vi "dropdown2.vi"(0 "side":enum16{"l", "r"}(ring), 1 "Boolean":bool) -> ()   [LabVIEW 2017]
uses:
  <vilib>/myRIO/Instrument Drivers/Onboard IO/DIO/typedefs/DIO Reference.ctl
  <vilib>/myRIO/Common/Instrument Driver Framework/Utilities/typedefs/myRIO Generic Hardware Reference.ctl
  <vilib>/myRIO/Common/Instrument Driver Framework/Utilities/typedefs/Hardware Version Enum.ctl
  <vilib>/myRIO/Common/Instrument Driver Framework/Utilities/typedefs/myRIO v1.0 Reference.ctl
  <vilib>/myRIO/Common/Instrument Driver Framework/Utilities/typedefs/Generic FPGA Reference.ctl
  <vilib>/myRIO/Common/Instrument Driver Framework/myRIO v1.0/DIO/typedefs/DIO Channels List.ctl
  <vilib>/myRIO/Common/Instrument Driver Framework/myRIO v1.0/DIO/typedefs/DIO Channels Enum.ctl
  <vilib>/userdefined/High Color/nirio_resource_hc.ctl
  <vilib>/myRIO/Common/Instrument Driver Framework/Utilities/vis/Is FPGA Ref Available.vi
  <vilib>/myRIO/Common/Instrument Driver Framework/myRIO v1.0/DIO/vis/myRIO v1.1 Open DIO.vi
  <vilib>/myRIO/Instrument Drivers/Onboard IO/DIO/vis/Read.vi
  <vilib>/myRIO/Common/Instrument Driver Framework/Utilities/vis/Validate Channels.vi
  <vilib>/myRIO/Common/Instrument Driver Framework/myRIO v1.0/DIO/vis/myRIO v1.0 Reserve DIO.vi
  <vilib>/myRIO/Common/Instrument Driver Framework/myRIO v1.0/Resource Manager/vis/myRIO v1.0 Reserve Channel List.vi
  <vilib>/myRIO/Common/Instrument Driver Framework/myRIO v1.0/DIO/vis/myRIO v1.0 Build MUX Configuration DIO.vi
  <vilib>/myRIO/Common/Instrument Driver Framework/myRIO v1.0/Resource Manager/vis/myRIO v1.0 Reserve Channel.vi
  <vilib>/myRIO/Common/Instrument Driver Framework/myRIO v1.0/Resource Manager/vis/myRIO v1.0 Unreserve Channel.vi
  <vilib>/myRIO/Common/Instrument Driver Framework/myRIO v1.0/Resource Manager/vis/myRIO v1.0 Create Configuration List.vi
  <vilib>/myRIO/Common/Instrument Driver Framework/myRIO v1.0/Resource Manager/vis/myRIO v1.0 Build Mutex Name.vi
  <vilib>/Utility/VariantDataType/GetNumericInfo.vi
  <vilib>/Utility/error.llb/Error Cluster From Error Code.vi
  <vilib>/myRIO/Common/Instrument Driver Framework/myRIO v1.0/myRIO v1.1 Open.vi
  <vilib>/myRIO/Common/Instrument Driver Framework/Utilities/vis/IO Manager.vi
  <vilib>/myRIO/Common/Instrument Driver Framework/Utilities/vis/Configuration Manager.vi
  <vilib>/myRIO/Common/Instrument Driver Framework/myRIO v1.0/Resource Manager/vis/myRIO v1.0 Configure IO.vi
  <vilib>/myRIO/Common/Instrument Driver Framework/myRIO v1.0/myRIO v1.0 Close.vi
  <vilib>/myRIO/Common/Instrument Driver Framework/myRIO v1.0/DIO/vis/myRIO v1.0 Read DIO.vi
  <vilib>/myRIO/Express VI/Onboard IO/DI/DI Express VI.xnode
  <vilib>/myRIO/Instrument Drivers/Onboard IO/DIO/vis/myRIO DIO Open.xnode
  <vilib>/myRIO/Instrument Drivers/Onboard IO/DIO/DIO.lvlib
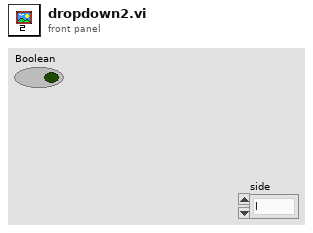
[diagram p1: front panel]
types:
  T1 = enum16{"hold", "f", "fl", "fr", "l", "r", "b", "bl", "br"}
  T2 = typedef "DIO.lvlib/DIO Reference.ctl" = cluster{"myRIO Reference":T3, "DIO Channels List":T7}
  T3 = typedef "myRIO Generic Hardware Reference.ctl" = cluster{"myRIO Model":T4, "myRIO Hardware Reference":T5}
  T4 = typedef "Hardware Version Enum.ctl" = enum16{"Unknown", "myRIO-1900", "myRIO-1950", "roboRIO", "NI ELVIS RIO CM"}
  T5 = typedef "myRIO v1.0 Reference.ctl" = cluster{"Generic FPGA Reference":T6, "Allow multiple opens":bool}
  T6 = typedef "Generic FPGA Reference.ctl" = refnum<k20>
  T7 = typedef "DIO Channels List.ctl" = T8[]
  T8 = typedef "DIO Channels Enum.ctl" = enum16{"Not Connected", "C/DIO0", "C/DIO1", "C/DIO2", "C/DIO3", "C/DIO4", "C/DIO5", "C/DIO6", "C/DIO7", "A/DIO0", "A/DIO1", "A/DIO2", "A/DIO3", "A/DIO4", "A/DIO5", "A/DIO6", "A/DIO7", "A/DIO8", "A/DIO9", "A/DIO10", "A/DIO11", "A/DIO12", "A/DIO13", "A/DIO14", "A/DIO15", "B/DIO0", "B/DIO1", "B/DIO2", "B/DIO3", "B/DIO4", "B/DIO5", "B/DIO6", "B/DIO7", "B/DIO8", "B/DIO9", "B/DIO10", "B/DIO11", "B/DIO12", "B/DIO13", "B/DIO14", "B/DIO15", "LED0", "LED1", "LED2", "LED3", "Button0", "DIO/DIO0", "DIO/DIO1", "DIO/DIO2", "DIO/DIO3", "DIO/DIO4", "DIO/DIO5", "DIO/DIO6", "DIO/DIO7", "DIO/DIO8", "DIO/DIO9", "SPI/CS0", "SPI/CS1", "SPI/CS2", "SPI/CS3", "LED RADIO (Green)", "LED RADIO (Red)", "LED COMM (Green)", "LED COMM (Red)", "LED MODE (Green)", "LED MODE (Red)"}
  T9 = typedef "nirio_resource_hc.ctl" = tag
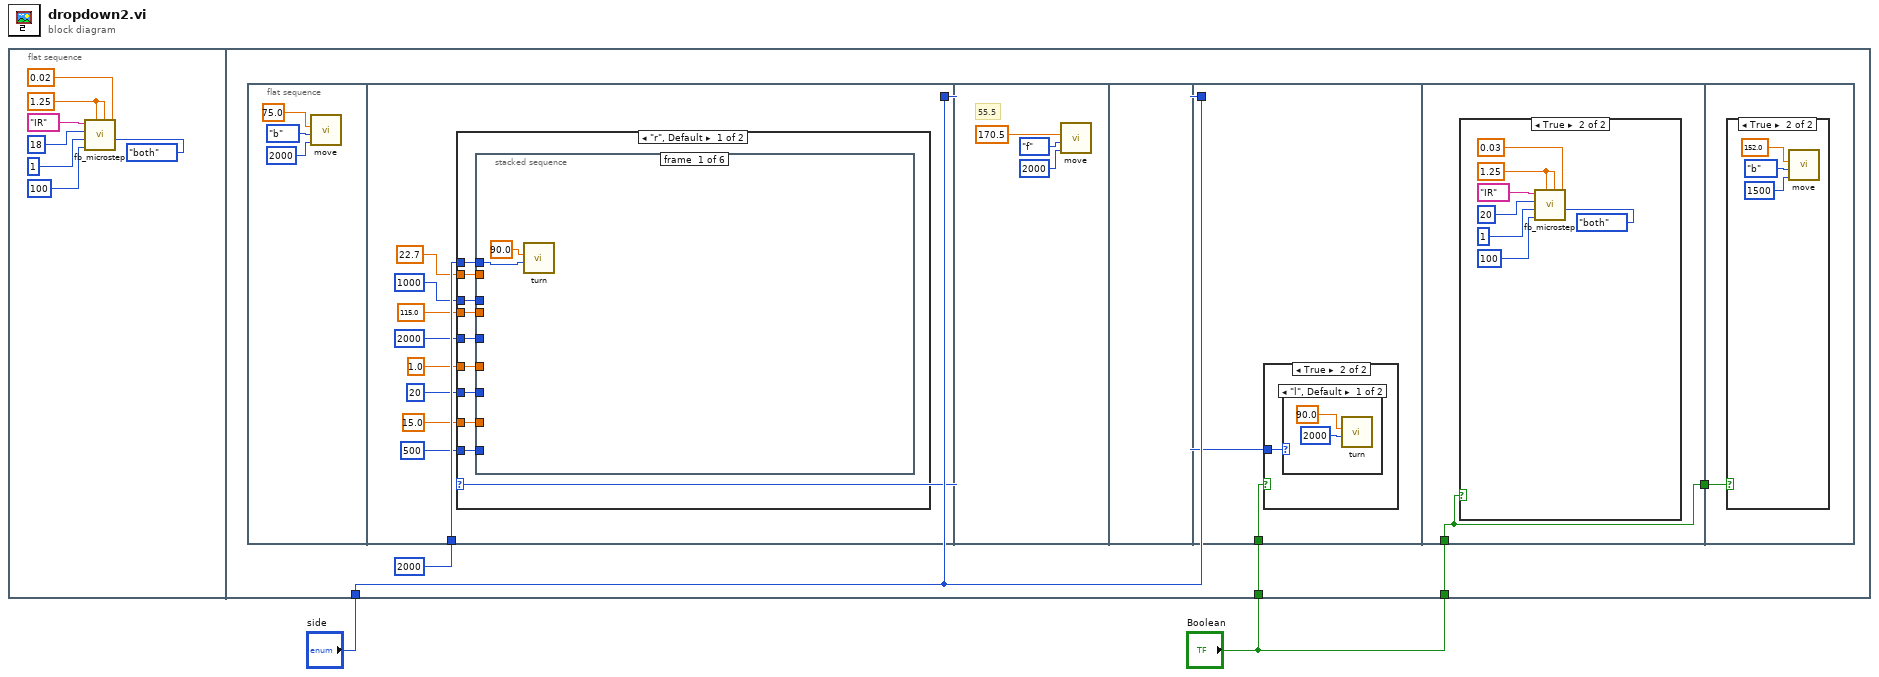
[diagram p0: block diagram]
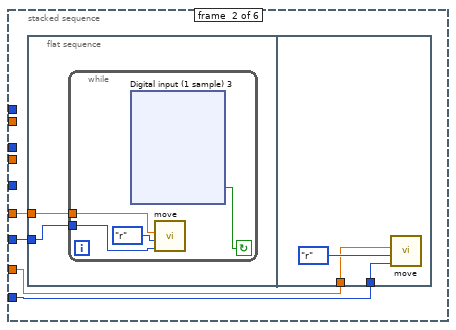
[diagram p2: hidden frame]
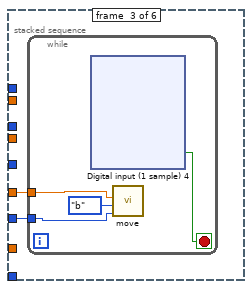
[diagram p3: hidden frame]
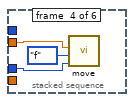
[diagram p4: hidden frame]
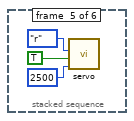
[diagram p5: hidden frame]
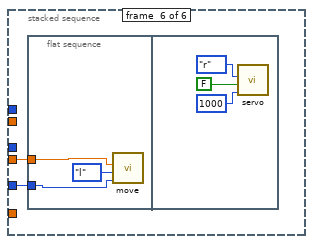
[diagram p6: hidden frame]
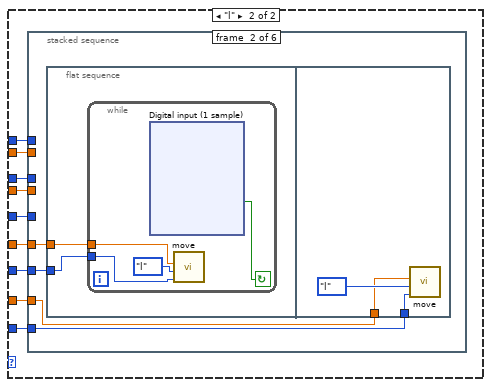
[diagram p7: hidden frame]
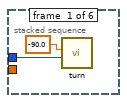
[diagram p8: hidden frame]
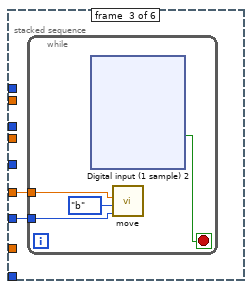
[diagram p9: hidden frame]
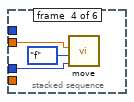
[diagram p10: hidden frame]
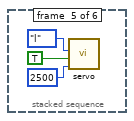
[diagram p11: hidden frame]
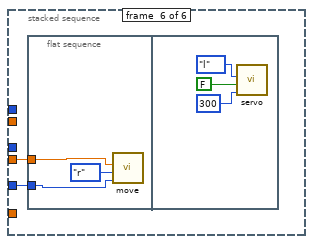
[diagram p12: hidden frame]
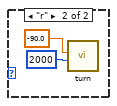
[diagram p14: hidden frame]
diagram:
  n1 = flat-sequence {
    tunnel: "side" -> [w13]
    tunnel: "Boolean" -> [w11]
    tunnel: "Boolean" -> [w10]
    frame #0 {
      w3 = 1.25 ("taget_IR_R")
      n2 = call "fb_microstep.vi"("Sensor"=enum16{"l", "r", "both"}."both", "precision"=0.02, "taget_IR_L"=w3, "taget_IR_R"=w3, "SamplingNUM"=100, "Step"=1, "Delay"=18, "Stop Mode"="IR") -> ()  [unwired: 3 in, 1 out]
    }
    frame #1 {
      n3 = flat-sequence {
        tunnel: w13 -> [w27]
        tunnel: u32 2000 ("delay") -> [w26]
        tunnel: w13 -> [w264]
        tunnel: w10 -> [w263]
        tunnel: [w270] -> w12
        tunnel: w11 -> [w270]
        tunnel: w12 -> [w278]
        frame #0 {
          n4 = call "move.vi"("delay"=u32 2000, "Enum"=T1."b", "D"=75.0) -> ()  [unwired: 9 in]
        }
        frame #1 {
          n5 = case shown="\"r\", Default" w27 {
            tunnel: w26 -> [w36 w152]
            tunnel: u32 20 ("delay") -> [w34 w151]
            tunnel: 1.0 ("D") -> [w35 w150]
            tunnel: 15.0 ("D") -> [w32 w149]
            tunnel: u32 500 ("delay") -> [w33 w148]
            tunnel: 22.7 ("D") -> [w31 w147]
            tunnel: u32 1000 ("delay") -> [w30 w146]
            tunnel: 115.0 ("D") -> [w29 w145]
            tunnel: u32 2000 ("delay") -> [w28 w144]
            frame "r", Default {
              n6 = stacked-sequence {
                tunnel: w36 -> [w37 _ _ _ _ _]
                tunnel: w35 -> [_ w42 w89 _ _ _]
                tunnel: w34 -> [_ w41 w88 _ _ _]
                tunnel: w33 -> [_ w40 _ _ _ _]
                tunnel: w32 -> [_ w39 _ _ _ _]
                tunnel: w31 -> [_ _ _ w131 _ _]
                tunnel: w30 -> [_ _ _ w130 _ _]
                tunnel: w29 -> [_ _ _ _ _ w137]
                tunnel: w28 -> [_ _ _ _ _ w136]
                frame #0 {
                  n7 = call "turn.vi"("delay"=w37, "Carzeta"=90.0) -> ()  [unwired: 10 in]
                }
                frame #1 {
                  n8 = flat-sequence {
                    tunnel: w42 -> [w44]
                    tunnel: w41 -> [w43]
                    tunnel: w40 -> [w86]
                    tunnel: w39 -> [w85]
                    frame #0 {
                      n9 = while {
                        tunnel: w44 -> [w47]
                        tunnel: w43 -> [w46]
                        stop <- w45 continue-if-true
                        n10 = xnode "Digital input (1 sample) 3"() -> ("R (A/DIO1 (Pin 13))"=w45:bool)  [unwired: 1 in, 2 out]
                        n11 = call "move.vi"("delay"=w46, "Enum"=T1."r", "D"=w47) -> ()  [unwired: 9 in]
                      }
                    }
                    frame #1 {
                      n12 = call "move.vi"("delay"=w86, "Enum"=T1."r", "D"=w85) -> ()  [unwired: 9 in]
                    }
                  }
                }
                frame #2 {
                  n13 = while {
                    tunnel: w89 -> [w92]
                    tunnel: w88 -> [w91]
                    stop <- w90 stop-if-true
                    n14 = xnode "Digital input (1 sample) 4"() -> ("R (A/DIO1 (Pin 13))"=w90:bool)  [unwired: 1 in, 2 out]
                    n15 = call "move.vi"("delay"=w91, "Enum"=T1."b", "D"=w92) -> ()  [unwired: 9 in]
                  }
                }
                frame #3 {
                  n16 = call "move.vi"("delay"=w130, "Enum"=T1."f", "D"=w131) -> ()  [unwired: 9 in]
                }
                frame #4 {
                  n17 = call "servo.vi"("delay"=u32 2500, "in=true\nout = false"=TRUE ("in=true\nout = false"), "left-right"=enum16{"r", "l"}."r") -> ()  [unwired: 9 in]
                }
                frame #5 {
                  n18 = flat-sequence {
                    tunnel: w137 -> [w139]
                    tunnel: w136 -> [w138]
                    frame #0 {
                      n19 = call "move.vi"("delay"=w138, "Enum"=T1."l", "D"=w139) -> ()  [unwired: 9 in]
                    }
                    frame #1 {
                      n20 = call "servo.vi"("delay"=u32 1000, "in=true\nout = false"=FALSE ("in=true\nout = false"), "left-right"=enum16{"r", "l"}."r") -> ()  [unwired: 9 in]
                    }
                  }
                }
              }
            }
            frame "l" {
              n21 = stacked-sequence {
                tunnel: w152 -> [w153 _ _ _ _ _]
                tunnel: w151 -> [_ w158 w205 _ _ _]
                tunnel: w150 -> [_ w157 w204 _ _ _]
                tunnel: w149 -> [_ w156 _ _ _ _]
                tunnel: w148 -> [_ w155 _ _ _ _]
                tunnel: w147 -> [_ _ _ w247 _ _]
                tunnel: w146 -> [_ _ _ w246 _ _]
                tunnel: w145 -> [_ _ _ _ _ w253]
                tunnel: w144 -> [_ _ _ _ _ w252]
                frame #0 {
                  n22 = call "turn.vi"("delay"=w153, "Carzeta"=-90.0) -> ()  [unwired: 10 in]
                }
                frame #1 {
                  n23 = flat-sequence {
                    tunnel: w158 -> [w160]
                    tunnel: w157 -> [w159]
                    tunnel: w156 -> [w202]
                    tunnel: w155 -> [w201]
                    frame #0 {
                      n24 = while {
                        tunnel: w160 -> [w162]
                        tunnel: w159 -> [w161]
                        stop <- w163 continue-if-true
                        n25 = xnode "Digital input (1 sample)"() -> ("L (A/DIO0 (Pin 11))"=w163:bool)  [unwired: 1 in, 2 out]
                        n26 = call "move.vi"("delay"=w162, "Enum"=T1."l", "D"=w161) -> ()  [unwired: 9 in]
                      }
                    }
                    frame #1 {
                      n27 = call "move.vi"("delay"=w201, "Enum"=T1."l", "D"=w202) -> ()  [unwired: 9 in]
                    }
                  }
                }
                frame #2 {
                  n28 = while {
                    tunnel: w205 -> [w207]
                    tunnel: w204 -> [w206]
                    stop <- w208 stop-if-true
                    n29 = xnode "Digital input (1 sample) 2"() -> ("L (A/DIO0 (Pin 11))"=w208:bool)  [unwired: 1 in, 2 out]
                    n30 = call "move.vi"("delay"=w207, "Enum"=T1."b", "D"=w206) -> ()  [unwired: 9 in]
                  }
                }
                frame #3 {
                  n31 = call "move.vi"("delay"=w246, "Enum"=T1."f", "D"=w247) -> ()  [unwired: 9 in]
                }
                frame #4 {
                  n32 = call "servo.vi"("delay"=u32 2500, "in=true\nout = false"=TRUE ("in=true\nout = false"), "left-right"=enum16{"r", "l"}."l") -> ()  [unwired: 9 in]
                }
                frame #5 {
                  n33 = flat-sequence {
                    tunnel: w253 -> [w255]
                    tunnel: w252 -> [w254]
                    frame #0 {
                      n34 = call "move.vi"("delay"=w254, "Enum"=T1."r", "D"=w255) -> ()  [unwired: 9 in]
                    }
                    frame #1 {
                      n35 = call "servo.vi"("delay"=u32 300, "in=true\nout = false"=FALSE ("in=true\nout = false"), "left-right"=enum16{"r", "l"}."l") -> ()  [unwired: 9 in]
                    }
                  }
                }
              }
            }
          }
        }
        frame #2 {
          # "55.5"
          n36 = call "move.vi"("delay"=u32 2000, "Enum"=T1."f", "D"=170.5) -> ()  [unwired: 9 in]
        }
        frame #3 {
        }
        frame #4 {
          n37 = case shown="True" w263 {
            tunnel: w264 -> [_ w265]
            frame False {
            }
            frame True {
              n38 = case shown="\"l\", Default" w265 {
                frame "l", Default {
                  n39 = call "turn.vi"("delay"=u32 2000, "Carzeta"=90.0) -> ()  [unwired: 10 in]
                }
                frame "r" {
                  n40 = call "turn.vi"("delay"=u32 2000, "Carzeta"=-90.0) -> ()  [unwired: 10 in]
                }
              }
            }
          }
        }
        frame #5 {
          n41 = case shown="True" w270 {
            frame False {
            }
            frame True {
              w271 = 1.25 ("taget_IR_R")
              n42 = call "fb_microstep.vi"("Sensor"=enum16{"l", "r", "both"}."both", "precision"=0.03, "taget_IR_L"=w271, "taget_IR_R"=w271, "SamplingNUM"=100, "Step"=1, "Delay"=20, "Stop Mode"="IR") -> ()  [unwired: 3 in, 1 out]
            }
          }
        }
        frame #6 {
          n43 = case shown="True" w278 {
            frame False {
            }
            frame True {
              n44 = call "move.vi"("delay"=u32 1500, "Enum"=T1."b", "D"=152.0) -> ()  [unwired: 9 in]
            }
          }
        }
      }
    }
  }
